vi "Flatten Value.vi"(8 "error in":errorcluster, 11 "2D String In":refnum<class "2D String.lvclass">) -> (0 "error out":errorcluster, 1 "Value":string, 3 "2D String Out":refnum<class "2D String.lvclass">)   [LabVIEW 2020, in "NI_VIAnCFGDataStructure.lvlib" / "2D String.lvclass"]
doc: "Dynamic dispatch interface for flattening Tree Data classes to string."
uses:
  <vilib>/addons/analyzer/VIAnCFGDataStructure/Data Types/2D String/2D String.lvclass
  <vilib>/addons/analyzer/VIAnCFGDataStructure/Data Types/2D String/2D String.lvclass/2D String.ctl
  <vilib>/addons/analyzer/VIAnCFGDataStructure/Tree Manager/API/Generate Hash.vi
  <vilib>/addons/analyzer/VIAnCFGDataStructure/Tree Manager/Tree.lvclass
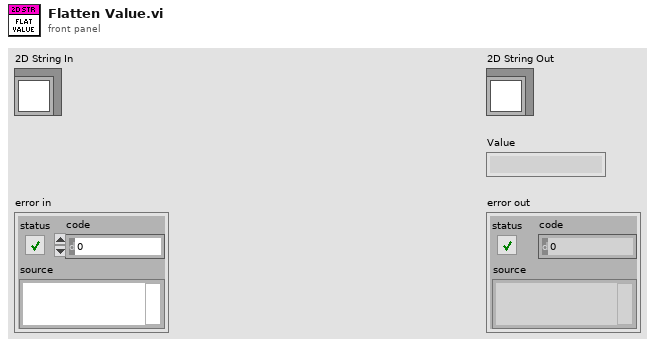
[diagram p1: front panel]
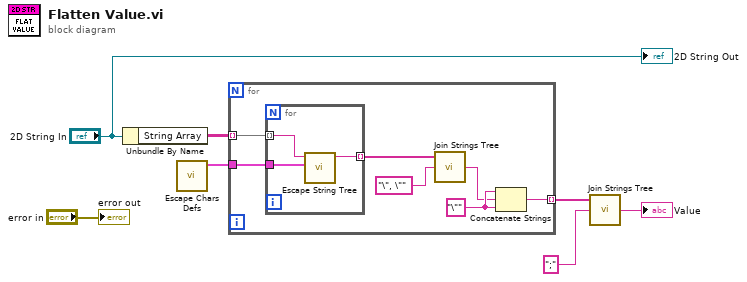
[diagram p0: block diagram]
diagram:
  n1 = Unbundle By Name("2D String In") -> ("String Array"=w7:string[][])
  n2 = call <vilib>:"Escape Chars Defs.vi"() -> ("Escapes"=w1:cluster{"String":string, "Escape":string}[])  [unwired: 11 in]
  n3 = for {
    tunnel: w7 -> [w13] mode=indexing
    tunnel: [w8] -> w6 mode=indexing
    tunnel: w1 -> [w14]
    w11 = "\"" ("string")
    n4 = for {
      tunnel: w14 -> [w16]
      tunnel: w13 -> [w17] mode=indexing
      tunnel: [w15] -> w9 mode=indexing
      n5 = call <vilib>:"Escape String Tree.vi"("Escapes"=w16, "String In"=w17) -> ("String Out"=w15:string)  [unwired: 9 in]
    }
    n6 = call <vilib>:"Join Strings Tree.vi"("Separator (,)"="\", \"", "Strings In"=w9) -> ("String"=w10:string)  [unwired: 1 in]
    n7 = Concatenate Strings(w11, w10, w11) -> (w8:string)
  }
  n8 = call <vilib>:"Join Strings Tree.vi"("Separator (,)"=";", "Strings In"=w6) -> ("String"=→"Value":string)  [unwired: 1 in]
  "2D String Out" <- "2D String In"
  "error out" <- "error in"
